vi "Timestamp to ISO8601 Date.vi"(9 "UTC? (F)":bool, 11 "Timestamp (now)":timestamp) -> (2 "ISO8601 Calendar Month":string, 3 "ISO8601 Date":string)   [LabVIEW 2017]
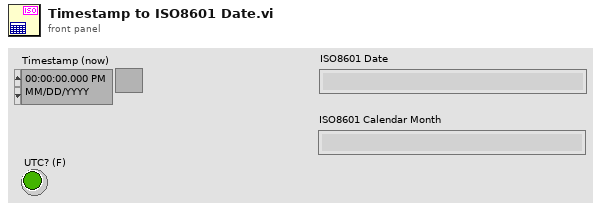
[diagram p1: front panel]
types:
  T1 = typedef "LVDateTimeRec.ctl" = cluster{"fractional second":dbl, "second":i32, "minute":i32, "hour":i32, "day of month":i32, "month":i32, "year":i32, "day of week":i32, "day of year":i32, "DST":i32}
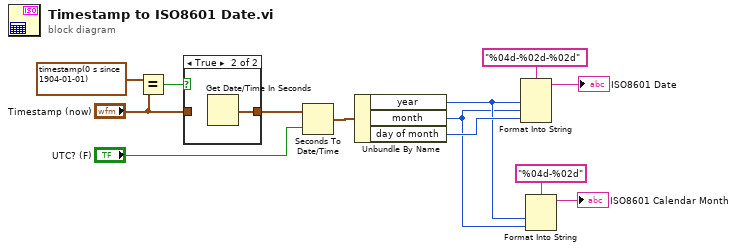
[diagram p0: block diagram]
diagram:
  n1 = Equal?(x=timestamp(0 s since 1904-01-01), y="Timestamp (now)") -> (x = y?=w7:bool)
  n2 = case shown="True" w7 {
    tunnel: [w14 w15] -> w5
    tunnel: "Timestamp (now)" -> [w14 _]
    frame False {
    }
    frame True {
      n3 = Get Date/Time In Seconds() -> (seconds since 1Jan1904=w15:timestamp)
    }
  }
  n4 = Seconds To Date/Time(time stamp (now)=w5, to UTC (F)="UTC? (F)") -> (date time rec=w10:T1)
  n5 = Unbundle By Name(w10) -> ("year"=w2:i32, "month"=w1:i32, "day of month"=w9:i32)
  n6 = Format Into String(format string="%04d-%02d-%02d", w2, w1, w9) -> (resulting string=→"ISO8601 Date":string)  [unwired: 2 in, 1 out]
  n7 = Format Into String(format string="%04d-%02d", w2, w1) -> (resulting string=→"ISO8601 Calendar Month":string)  [unwired: 2 in, 1 out]
